vi "Send Set Loop Period Msg.vi"(8 "error in (no error)":errorcluster, 10 "Loop Period in ms (10)":u32=10, 11 "Message Queue in":refnum<queue>) -> (0 "error out":errorcluster, 3 "Message Queue out":refnum<queue>)   [LabVIEW 2024, in "PID Loop.lvlib" / "Set Loop Period Msg.lvclass"]
uses:
  Set Loop Period Msg.lvclass
  Set Loop Period Msg.lvclass/Set Loop Period Msg.ctl
  C:/Users/uspoaotto/OneDrive - Oregon Tool/Desktop/working copies/zeroTimeoutMessageHandler/samples/PID Controller/PID Loop/PID Loop/Set Loop Period Msg/Set Loop Period Msg.lvclass
  C:/Users/uspoaotto/OneDrive - Oregon Tool/Desktop/working copies/zeroTimeoutMessageHandler/src/Zero Timeout Message Handler/~Message/~Message.lvclass
  src/Zero Timeout Message Handler/~Message/~Message.lvclass
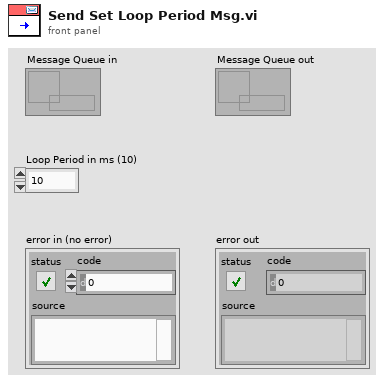
[diagram p1: front panel]
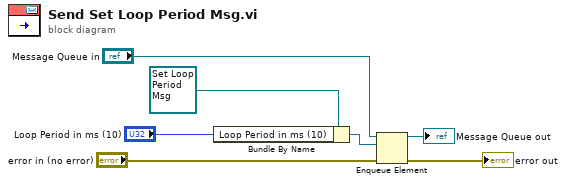
[diagram p0: block diagram]
diagram:
  n1 = Bundle By Name(cluster=refnum<class "Set Loop Period Msg.lvclass"> refnum ("PID Loop.lvlib:Set Loop Period Msg.lvclass"), "Loop Period in ms (10)"="Loop Period in ms (10)") -> (w4:refnum<class "Set Loop Period Msg.lvclass">)
  n2 = Enqueue Element(queue="Message Queue in", element=w4, error in (no error)="error in (no error)") -> (queue out=→"Message Queue out":refnum<queue>, error out=→"error out":errorcluster)  [unwired: 1 in, 1 out]
